vi "readNotifierServerStatus.vi"(8 "error in (no error)":errorcluster, 9 "notifierStatusOld":bool, 10 "serverSelection":enum16{"cmd", "tel"}(ring), 11 "TcpServer in":refnum<class "TcpServer.lvclass">) -> (0 "error out (no error)":errorcluster, 1 "notifierStatusNew":bool, 3 "TcpServer out":refnum<class "TcpServer.lvclass">)   [LabVIEW 2018, in "TcpServer.lvclass"]
doc: "Read the notifierServerStatus sent from tcpServerStateMachine.vi.\n\nNotes: \n1. Put this VI in Prealocated reentrant clone execution.\n2. This vi is public for test purspose only. Please don´t use this vi."
uses:
  TcpServer.lvclass
  TcpServer.lvclass/TcpServer.ctl
  TcpServerBase/TcpServerBase.lvclass/TcpServerBase.ctl
  TcpServerCmd/TcpServerCmd.lvclass
  home/pcortes/Documents/github/ts_labview_tcp_json/src/TcpServerBase/TcpServerBase.lvclass
  TcpServerTel/TcpServerTel.lvclass
  TcpServerBase/TcpServerBase.lvclass
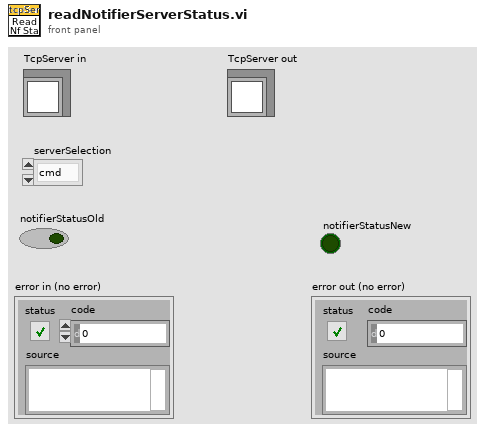
[diagram p1: front panel]
types:
  T1 = cluster{"connectionStatus":bool, "errorSource":string}
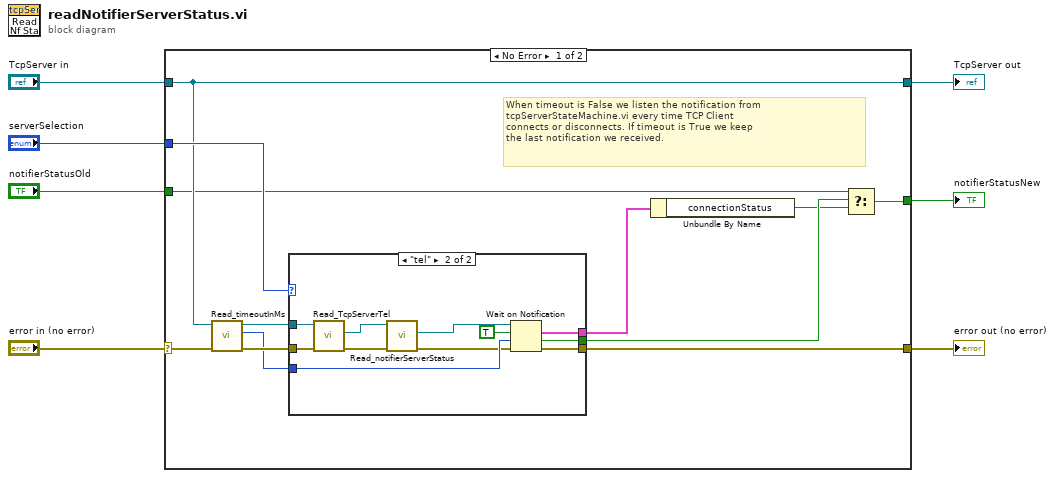
[diagram p0: block diagram]
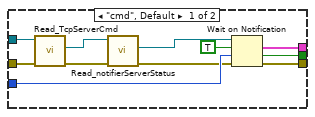
[diagram p2: hidden frame]
diagram:
  n1 = case shown="No Error" "error in (no error)" {
    selector: "error in (no error)" -> [w18 w43]
    tunnel: [w8 w44] -> w7
    tunnel: "notifierStatusOld" -> [w9 w44]
    tunnel: [w12 w43] -> w4
    tunnel: [w14 w42] -> w2
    tunnel: "TcpServer in" -> [w14 w42]
    tunnel: "serverSelection" -> [w19 _]
    frame No Error {
      # "When timeout is False we listen the notification from\ntcpServerStateMachine.vi every time TCP Client\nconnects or disconnects. If timeout is True we keep\nthe last notification we received."
      n2 = call "Read_timeoutInMs.vi"("error in (no error)"=w18, "TcpServer in"=w14) -> ("error out"=w17:errorcluster, "timeoutInMs"=w15:i32, "TcpServer out"=w16:refnum<class "TcpServer.lvclass">)  [unwired: 7 in]
      n3 = case shown="\"tel\"" w19 {
        tunnel: w17 -> [w29 w41]
        tunnel: w16 -> [w30 w40]
        tunnel: w15 -> [w26 w35]
        tunnel: [w25 w36] -> w13
        tunnel: [w24 w37] -> w11
        tunnel: [w23 w38] -> w12
        frame "cmd", Default {
          n4 = call "Read_TcpServerCmd.vi"("error in (no error)"=w29, "TcpServer in"=w30) -> ("error out"=w28:errorcluster, "TcpServerCmd.lvclass"=w27:refnum<class "TcpServerCmd.lvclass">)  [unwired: 7 in, 1 out]
          n5 = call "Read_notifierServerStatus.vi"("error in (no error)"=w28, "TcpServerBase in"=w27) -> ("error out"=w21:errorcluster, "notifierServerStatus"=w22:refnum<notifier>)  [unwired: 7 in, 1 out]
          n6 = Wait on Notification(notifier=w22, ignore previous (F)=TRUE, timeout in ms (-1)=w26, error in (no error)=w21) -> (notification=w25:T1, timed out?=w24:bool, error out=w23:errorcluster)  [unwired: 1 out]
        }
        frame "tel" {
          n7 = call "Read_TcpServerTel.vi"("error in (no error)"=w41, "TcpServer in"=w40) -> ("error out"=w39:errorcluster, "TcpServerTel.lvclass"=w34:refnum<class "TcpServerTel.lvclass">)  [unwired: 7 in, 1 out]
          n8 = call "Read_notifierServerStatus.vi"("error in (no error)"=w39, "TcpServerBase in"=w34) -> ("error out"=w33:errorcluster, "notifierServerStatus"=w32:refnum<notifier>)  [unwired: 7 in, 1 out]
          n9 = Wait on Notification(notifier=w32, ignore previous (F)=TRUE, timeout in ms (-1)=w35, error in (no error)=w33) -> (notification=w36:T1, timed out?=w37:bool, error out=w38:errorcluster)  [unwired: 1 out]
        }
      }
      n10 = Unbundle By Name(w13) -> ("connectionStatus"=w10:bool)
      n11 = Select(t=w9, s=w11, f=w10) -> (s? t:f=w8:bool)
    }
    frame Error {
    }
  }
  "notifierStatusNew" <- w7
  "error out (no error)" <- w4
  "TcpServer out" <- w2
